vi "Calculate IQ Power Level.vi"(0 "IQ data":cdb[](array[numeric])) -> (4 "power level (dBm)":dbl[](array[numeric]))   [LabVIEW 2017]
doc: "Calculate the IQ power level based on the IQ data.\n\n<B>Input Parameters</B>\n\n<B>IQ data</B> is the input.\n\n<B>Output Parameters</B>\n\n<B>power level (dBm)</B> is the power level for the IQ data input."
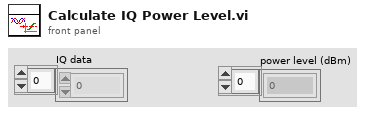
[diagram p1: front panel]
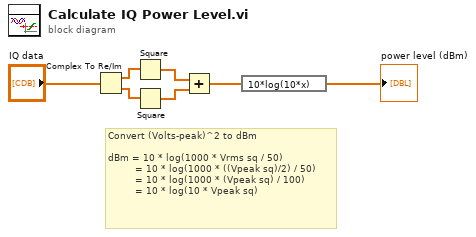
[diagram p0: block diagram]
diagram:
  # "Convert (Volts-peak)^2 to dBm\n\ndBm = 10 * log(1000 * Vrms sq / 50)\n         = 10 * log(1000 * ((Vpeak sq)/2) / 50) \n         = 10 * log(1000 * (Vpeak sq) / 100) \n         = 10 * log(10 * Vpeak sq)"
  n1 = Complex To Re/Im(x + iy="IQ data") -> (x=w6:dbl[], y=w5:dbl[])
  n2 = Square(x=w6) -> (x^2=w4:dbl[])
  n3 = Square(x=w5) -> (x^2=w3:dbl[])
  n4 = Add(x=w4, y=w3) -> (x+y=w2:dbl[])
  n5 = expression code="10*log(10*x)"(w2) -> (→"power level (dBm)":dbl[])
